vi "Write Temperature Range.vi"(8 "error in (no error)":errorcluster, 11 "Cooler in":refnum<class "Cooler.lvclass">) -> (0 "error out":errorcluster, 3 "Cooler out":refnum<class "Cooler.lvclass">)   [LabVIEW 2018, in "Cooler.lvclass"]
uses:
  Cooler.lvclass
  Cooler.lvclass/Cooler.ctl
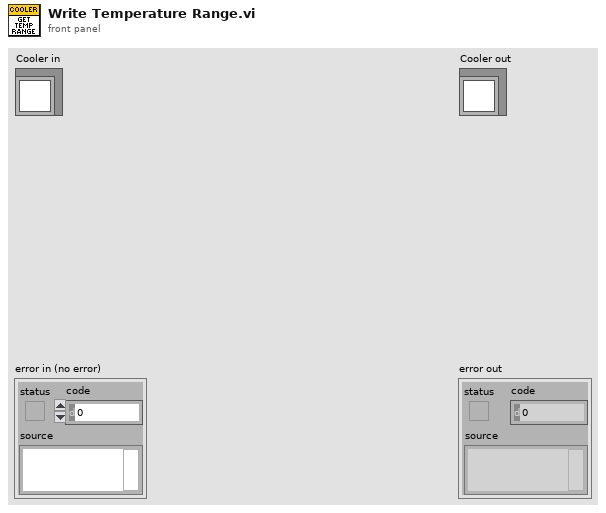
[diagram p1: front panel]
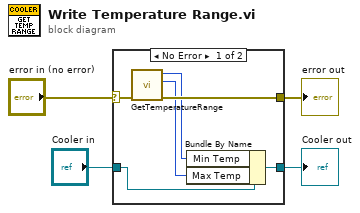
[diagram p0: block diagram]
diagram:
  n1 = case shown="No Error" "error in (no error)" {
    selector: "error in (no error)" -> [w10 w12]
    tunnel: [w9 w12] -> w2
    tunnel: [w5 w11] -> w1
    tunnel: "Cooler in" -> [w8 w11]
    frame No Error {
      n2 = call <userlib>:"GetTemperatureRange.vi"("error in (no error)"=w10) -> ("error out"=w9:errorcluster, "maxTemp"=w6:i32, "minTemp"=w7:i32)  [unwired: 3 in, 1 out]
      n3 = Bundle By Name(cluster=w8, "Min Temp"=w7, "Max Temp"=w6) -> (w5:refnum<class "Cooler.lvclass">)
    }
    frame Error {
    }
  }
  "error out" <- w2
  "Cooler out" <- w1
